vi "Shutdown Status.vi"(8 "error in":errorcluster, 11 "FPGA VI Reference In":T1) -> (0 "error out":errorcluster, 2 "Subsystem Status":T2, 3 "FPGA VI Reference Out":T1)   [LabVIEW 2015]
uses:
  Subsystem Status.ctl
  Subsystem Status Severity.ctl
  Subsystem Status Message.ctl
  FPGA Typedef.ctl
  AIR Status.ctl
  <vilib>/Utility/error.llb/Error Cluster From Error Code.vi
  <vilib>/rvi/errors/niLvFpgaAdjustHostInterfaceError.vi
  Global Data.vi
  <vilib>/rvi/interface/nirviReadWriteControl/nirviReadWriteControl.xnode
  FPGA Bitfiles/Latest.lvbitx
  NiFpgaLv.dll
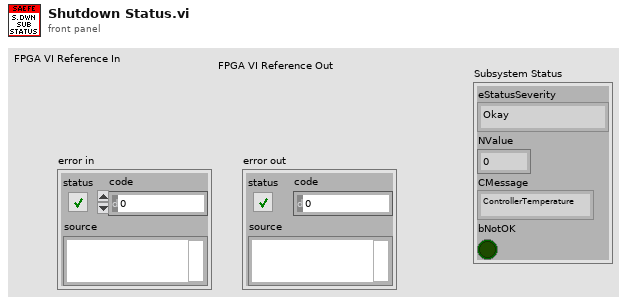
[diagram p1: front panel]
types:
  T1 = typedef "FPGA Typedef.ctl" = refnum<k20>
  T2 = typedef "Subsystem Status.ctl" = cluster{"eStatusSeverity":T3, "NValue":sgl, "CMessage":T4, "bNotOK":bool}
  T3 = typedef "Subsystem Status Severity.ctl" = enum16{"Okay", "Short Warning", "Long Warning", "Return to Pits", "Error", "Danger"}
  T4 = typedef "Subsystem Status Message.ctl" = enum16{"ControllerTemperature", "MotorTemperature", "BatteryTemperature", "BatteryLowVoltage", "LVBattery", "sbRIOTemperature", "Precharge", "BSPD", "IMD", "RemoteReturnToPits", "EStopInterrupted", "NoCellComms", "MCOverSpeed", "MCOverCurrent", "MCOverVoltage", "MCInverterOverTemp", "MCDirectionCommand", "MCInverterTimeout", "MCDesatFault", "MCHWOverCurrent", "MCUnderVoltage", "MCCommandMessageLost", "MotorOverTemp", "MCModAOverTemp", "MCModBOverTemp", "MCModCOverTemp", "MCPCBOverTemp", "MCGateDrv1OverTemp", "MCDateDrv2OverTemp", "MCCurrentSensorFault", "MCResolverNotConnected", "ShutdownLatchTripped", "UnknownBMS", "RemoteEmergency"}
  T5 = typedef "AIR Status.ctl" = enum16{"Off", "Precharge", "On"}
  T6 = typedef "MC Voltage.ctl" = cluster{"VMCPhaseAB":dbl, "VMCPhaseBC":dbl, "VMCOutput":dbl, "VMCBattery":dbl}
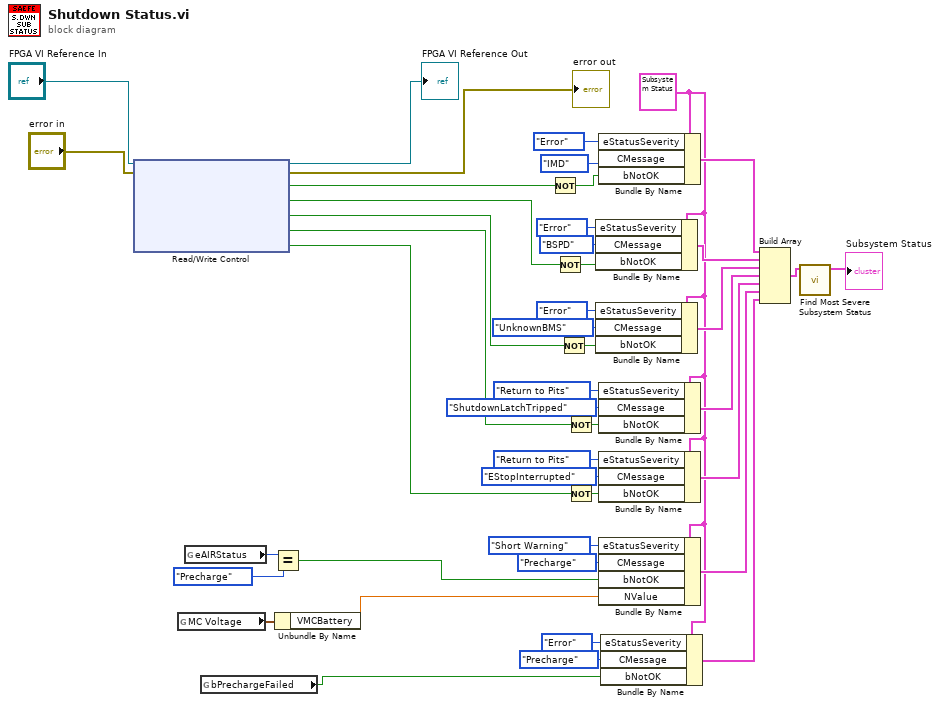
[diagram p0: block diagram]
diagram:
  w7 = T2 {"eStatusSeverity"=enum."Okay", "NValue"=0.0, "CMessage"=enum."ControllerTemperature", "bNotOK"=FALSE} ("Subystem Status")
  n1 = xnode "Read/Write Control"("FPGA VI Reference In"="FPGA VI Reference In", "error in"="error in") -> ("FPGA VI Reference Out"=→"FPGA VI Reference Out":T1, "error out"=→"error out":errorcluster, "bIMDOK"=w3:bool, "bBSPDOK"=w2:bool, "bBMSOK"=w1:bool, "bTSMSOutStatus"=w30:bool, "bTSMSInStatus"=w24:bool)
  n2 = global read "Global Data.vi" "MC Voltage"() -> (w5:T6)
  n3 = global read "Global Data.vi" "eAIRStatus"() -> (w16:T5)
  n4 = global read "Global Data.vi" "bPrechargeFailed"() -> (w6:bool)
  n5 = Equal?(x=w16, y=AIR_Status."Precharge") -> (x = y?=w11:bool)
  n6 = Unbundle By Name(w5) -> ("VMCBattery"=w4:dbl)
  n7 = Not(x=w3) -> (.not. x?=w34:bool)
  n8 = Not(x=w2) -> (.not. x?=w35:bool)
  n9 = Not(x=w1) -> (.not. x?=w36:bool)
  n10 = Not(x=w30) -> (.not. x?=w31:bool)
  n11 = Not(x=w24) -> (.not. x?=w27:bool)
  n12 = Bundle By Name(cluster=w7, "eStatusSeverity"=Subsystem_Status_Severity."Error" ("Status Severity"), "CMessage"=Subsystem_Status_Message."BSPD" ("Message"), "bNotOK"=w35) -> (w22:T2)
  n13 = Bundle By Name(cluster=w7, "eStatusSeverity"=Subsystem_Status_Severity."Error" ("Status Severity"), "CMessage"=Subsystem_Status_Message."UnknownBMS" ("Message"), "bNotOK"=w36) -> (w21:T2)
  n14 = Bundle By Name(cluster=w7, "eStatusSeverity"=Subsystem_Status_Severity."Error" ("Status Severity"), "CMessage"=Subsystem_Status_Message."IMD" ("Message"), "bNotOK"=w34) -> (w23:T2)
  n15 = Bundle By Name(cluster=w7, "eStatusSeverity"=Subsystem_Status_Severity."Return to Pits" ("Status Severity"), "CMessage"=Subsystem_Status_Message."ShutdownLatchTripped" ("Message"), "bNotOK"=w31) -> (w20:T2)
  n16 = Bundle By Name(cluster=w7, "eStatusSeverity"=Subsystem_Status_Severity."Return to Pits" ("Status Severity"), "CMessage"=Subsystem_Status_Message."EStopInterrupted" ("Message"), "bNotOK"=w27) -> (w19:T2)
  n17 = Bundle By Name(cluster=w7, "eStatusSeverity"=Subsystem_Status_Severity."Short Warning" ("Status Severity"), "CMessage"=Subsystem_Status_Message."Precharge" ("Message"), "bNotOK"=w11, "NValue"=w4) -> (w12:T2)
  n18 = Bundle By Name(cluster=w7, "eStatusSeverity"=Subsystem_Status_Severity."Error" ("Status Severity"), "CMessage"=Subsystem_Status_Message."Precharge" ("Message"), "bNotOK"=w6) -> (w8:T2)
  n19 = Build Array(w23, w22, w21, w20, w19, w12, w8) -> (w18:T2[])
  n20 = call "Find Most Severe Subsystem Status.vi"("Array"=w18) -> ("Subystem Status"=→"Subsystem Status":T2)  [unwired: 10 in]
